vi "Noise Generation.vi"() -> ()   [LabVIEW 2019]
doc: "Generates a monotone signal. If you are setting up a demo system of active noise control, you can use this VI to simulate a noisy environment with monotone noise."
uses:
  <vilib>/sound2/lvsound2.llb/Sampling Mode.ctl
  <vilib>/sound2/lvsound2.llb/Sound Data Format.ctl
  <vilib>/sound2/lvsound2.llb/Sound Output Set Volume (Single).vi
  <vilib>/sound2/lvsound2.llb/Sound Output Write (DBL).vi
  <vilib>/measure/NI_MABase.lvlib
panel:
  in  "tones":T1(array[cluster])=[{"frequency"=120.0, "amplitude"=0.4, "phase"=0.0}, {"frequency"=240.0, "amplitude"=0.3, "phase"=0.0}, {"frequency"=360.0, "amplitude"=0.5, "phase"=0.0}] {"phase" format="%.2p"; "amplitude" format="%0.2p"; "frequency" format="%0.2p"}
  in  "Stop":bool
  # "Monotone Noise Generation"
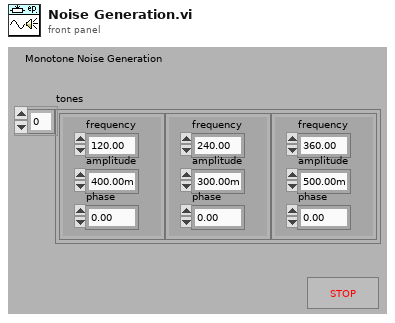
[diagram p1: front panel]
types:
  T1 = cluster{"frequency":dbl, "amplitude":dbl, "phase":dbl}[]
  T2 = typedef "Sound Data Format.ctl" = cluster{"sample rate (S/s)":dbl, "number of channels":i32, "bits per sample":i32}
  T3 = typedef "Sampling Mode.ctl" = i32
  T4 = typedef "Sound Output Task ID.ctl" = u32
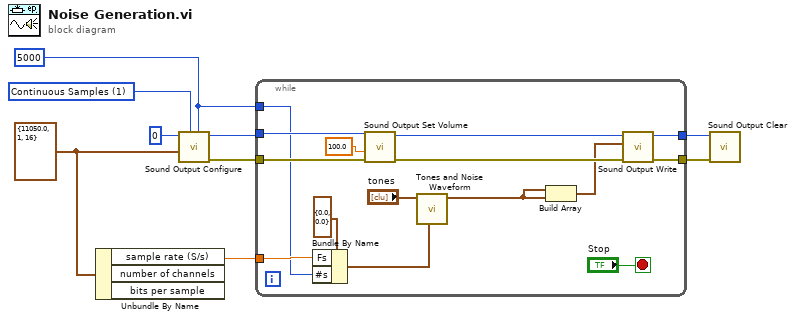
[diagram p0: block diagram]
diagram:
  w4 = T2 {"sample rate (S/s)"=11050.0, "number of channels"=1, "bits per sample"=16} ("sound format")
  w2 = 5000 ("number of samples/ch")
  w1 = T3 1 items=["Finite Samples", "Continuous Samples"] ("sample mode")
  n1 = Unbundle By Name(w4) -> ("sample rate (S/s)"=w3:dbl)  [unwired: 2 out]
  n2 = call <vilib>:"Sound Output Configure.vi"("number of samples/ch"=w2, "sample mode"=w1, "sound format"=w4, "device ID"=u32 0) -> ("error out"=w6:errorcluster, "task ID"=w8:T4)  [unwired: 1 in, 5 out]
  n3 = while {
    tunnel: w3 -> [w15]
    tunnel: w2 -> [w14]
    tunnel: w8 -> [w23]
    tunnel: [w21] -> w7
    tunnel: w6 -> [w20]
    tunnel: [w17] -> w5
    stop <- "Stop" stop-if-true
    n4 = Bundle By Name(cluster=cluster{"Fs":dbl, "#s":dbl} {"Fs"=0.0, "#s"=0.0} ("sampling info"), "Fs"=w15, "#s"=w14) -> (w12:cluster{"Fs":dbl, "#s":dbl})
    n5 = call-poly <vilib>:"Sound Output Set Volume.vi"("error in (no error)"=w20, "volume"=100.0, "task ID"=w23) -> ("error out"=w19:errorcluster, "task ID out"=w22:T4)  [unwired: 7 out]
    n6 = call <vilib>:"Tones and Noise Waveform.vi"("sampling info"=w12, "tones"="tones") -> ("signal out"=w10:waveform(dbl))  [unwired: 5 in, 4 out]
    n7 = Build Array(w10, w10) -> (w13:waveform(dbl)[])
    n8 = call-poly <vilib>:"Sound Output Write.vi"("error in (no error)"=w19, "data"=w13, "task ID"=w22) -> ("error out"=w17:errorcluster, "task ID out"=w21:T4)  [unwired: 1 in, 6 out]
  }
  n9 = call <vilib>:"Sound Output Clear.vi"("error in (no error)"=w5, "task ID"=w7) -> ()  [unwired: 10 out]
